vi "Get Ctl Reference.vi"(8 "error in":errorcluster, 11 "id":string) -> (0 "error out":errorcluster, 3 "ctl reference":refnum<vi>)   [LabVIEW 2020, in "G-AI Core.lvlib"]
uses:
  G-AI Core.lvlib
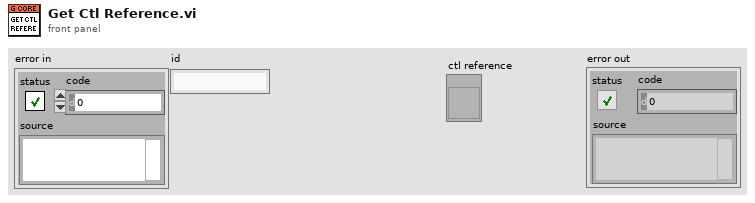
[diagram p1: front panel]
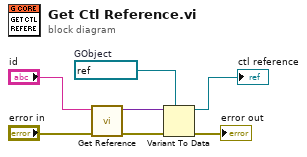
[diagram p0: block diagram]
diagram:
  w5 = refnum<vi> refnum  # GObject
  n1 = call "Get Reference.vi"("error in"="error in", "id"="id") -> ("error out"=w7:errorcluster, "reference"=w6:variant)  [unwired: 8 in]
  n2 = Variant To Data(error in=w7, type=w5, Variant=w6) -> (data=→"ctl reference":refnum<vi>, error out=→"error out":errorcluster)
